vi "Version_2.0_Single_Column_Code.vi"() -> ()   [LabVIEW 2020] (continued)
                            # "Clean the tubing with Sample"
                            n4641 = local read "N-S"() -> (w5076:i32)
                            n4642 = for {
                              N: w5076 -> [_]
                              n4643 = stacked-sequence {
                                frame #0 {
                                n4644 = local read "VISA Refnum in\nfor Pump"() -> (w5079:refnum<visa-resource-name>)
                                n4645 = local read "Port for \nSample"() -> (w5078:string)
                                n4646 = call "PortChanger (SubVI).vi"("Port Number"=w5078, "VISA Refnum in"=w5079) -> ()  [unwired: 10 in]
                                }
                                frame #1 {
                                n4647 = local read "VISA Refnum in\nfor Pump"() -> (w5080:refnum<visa-resource-name>)
                                n4648 = call "ProcessCompletionWaiter (SubVI).vi"("VISA Refnum in"=w5080) -> ()  [unwired: 11 in]
                                }
                                frame #2 {
                                n4649 = local read "VISA Refnum in\nfor Pump"() -> (w5085:refnum<visa-resource-name>)
                                n4650 = local read "Sample PickUp \nFlow Rate (ul/min)"() -> (w5082:dbl)
                                n4651 = local read "V-S"() -> (w5081:dbl)
                                n4652 = local read "Volume of Syringe"() -> (w5083:dbl)
                                n4653 = call "RPickUp(SubVI).vi"("Volume to be picked up"=w5081, "Volume of Syringe"=w5083, "Resolution of PickUP"=T2."Standard Pumping", "PickUp Flow Rate (ul/min)"=w5082, "VISA Refnum in"=w5085) -> ()  [unwired: 6 in, 1 out]
                                }
                                frame #3 {
                                n4654 = local read "Stopper that ends \nthe main loops"() -> (w5086:bool)
                                n4655 = local read "VISA Refnum in\nfor Pump"() -> (w5087:refnum<visa-resource-name>)
                                n4656 = case shown="True" w5086 {
                                frame False {
                                }
                                frame True {
                                n4657 = local read "VISA Refnum in\nfor Pump"() -> (w5088:refnum<visa-resource-name>)
                                n4658 = call "HardStopCurrentProcess (SubVI).vi"("VISA Refnum in"=w5088) -> ()  [unwired: 11 in]
                                }
                                }
                                n4659 = call "ProcessCompletionWaiter (SubVI).vi"("VISA Refnum in"=w5087) -> ()  [unwired: 11 in]
                                }
                                frame #4 {
                                n4660 = local read "VISA Refnum in\nfor Pump"() -> (w5090:refnum<visa-resource-name>)
                                n4661 = call "PortChanger (SubVI).vi"("Port Number"="1", "VISA Refnum in"=w5090) -> ()  [unwired: 10 in]
                                }
                                frame #5 {
                                n4662 = local read "Stopper that ends \nthe main loops"() -> (w5091:bool)
                                n4663 = local read "VISA Refnum in\nfor Pump"() -> (w5092:refnum<visa-resource-name>)
                                n4664 = case shown="True" w5091 {
                                frame False {
                                }
                                frame True {
                                n4665 = local read "VISA Refnum in\nfor Pump"() -> (w5093:refnum<visa-resource-name>)
                                n4666 = call "HardStopCurrentProcess (SubVI).vi"("VISA Refnum in"=w5093) -> ()  [unwired: 11 in]
                                }
                                }
                                n4667 = call "ProcessCompletionWaiter (SubVI).vi"("VISA Refnum in"=w5092) -> ()  [unwired: 11 in]
                                }
                                frame #6 {
                                n4668 = local read "VISA Refnum in\nfor Pump"() -> (w5098:refnum<visa-resource-name>)
                                n4669 = local read "Volume of Syringe"() -> (w5095:dbl)
                                n4670 = call "GoToAbsolutePosition(SubVI).vi"("Absolute Volume Position in Syringe (in ul)"=0.0 ("Volume to be picked up"), "Volume of Syringe"=w5095, "Resolution of Pumping"=T2."Standard Pumping" ("Resolution of PickUP"), "Flow Rate (ul/min)"=150.0 ("PickUp Flow Rate (ul/min)"), "VISA Refnum in"=w5098) -> ()  [unwired: 6 in, 1 out]
                                }
                                frame #7 {
                                n4671 = local read "Stopper that ends \nthe main loops"() -> (w5099:bool)
                                n4672 = local read "VISA Refnum in\nfor Pump"() -> (w5100:refnum<visa-resource-name>)
                                n4673 = case shown="True" w5099 {
                                frame False {
                                }
                                frame True {
                                n4674 = local read "VISA Refnum in\nfor Pump"() -> (w5101:refnum<visa-resource-name>)
                                n4675 = call "HardStopCurrentProcess (SubVI).vi"("VISA Refnum in"=w5101) -> ()  [unwired: 11 in]
                                }
                                }
                                n4676 = call "ProcessCompletionWaiter (SubVI).vi"("VISA Refnum in"=w5100) -> ()  [unwired: 11 in]
                                }
                              }
                              n4677 = local write "Pause Data Collection"(TRUE ("Pause Data Collection")) -> ()
                            }
                          }
                        }
                      }
                      frame #1 {
                        # "Pump Sample into Column-1"
                        n4678 = stacked-sequence {
                          frame #0 {
                            # "Switch to Port-3"
                            # "Port-3 of pump is connected to Sample"
                            n4679 = local read "VISA Refnum in\nfor Pump"() -> (w5106:refnum<visa-resource-name>)
                            n4680 = local read "Port for \nSample"() -> (w5105:string)
                            n4681 = call "PortChanger (SubVI).vi"("Port Number"=w5105, "VISA Refnum in"=w5106) -> ()  [unwired: 10 in]
                          }
                          frame #1 {
                            n4682 = local read "VISA Refnum in\nfor Pump"() -> (w5107:refnum<visa-resource-name>)
                            n4683 = call "ProcessCompletionWaiter (SubVI).vi"("VISA Refnum in"=w5107) -> ()  [unwired: 11 in]
                          }
                          frame #2 {
                            n4684 = local write "Valve V1 Open"(TRUE ("Valve V1 Open")) -> ()
                            n4685 = local write "Valve V2 Open"(TRUE ("Valve V2 Open")) -> ()
                            n4686 = local write "Valve V3 Open"(FALSE ("Valve V3 Open")) -> ()
                            n4687 = local write "Valve V4 Open"(FALSE ("Valve V4 Open")) -> ()
                            n4688 = local write "External Valve \nOpen"(TRUE ("External Valve \nOpen")) -> ()
                            n4689 = local write "Valve V5 Open"(FALSE ("Valve V5 Open")) -> ()
                            n4690 = local write "Valve V8 Open"(FALSE ("Valve V8 Open")) -> ()
                            n4691 = local write "Valve V6 Open"(FALSE ("Valve V6 Open")) -> ()
                            n4692 = local write "Valve V7 Open"(FALSE ("Valve V7 Open")) -> ()
                          }
                          frame #3 {
                            n4693 = local read "Apparent Volume\nof Syringe"() -> (w5117:dbl)
                            n4694 = local read "Sample Volume \nto be Pumped"() -> (w5120:dbl)
                            n4695 = Quotient & Remainder(x=w5120, y=w5117) -> (x-y*floor(x/y)=w5118:dbl, floor(x/y)=w5119:dbl)
                            n4696 = for {
                              N: w5119 -> [_]
                              n4697 = stacked-sequence {
                                frame #0 {
                                n4698 = local read "Sample PickUp \nFlow Rate (ul/min)"() -> (w5123:dbl)
                                n4699 = local read "Sample Pumping\nResolution"() -> (w5122:T2)
                                n4700 = local read "VISA Refnum in\nfor Pump"() -> (w5125:refnum<visa-resource-name>)
                                n4701 = local read "Apparent Volume\nof Syringe"() -> (w5121:dbl)
                                n4702 = local read "Volume of Syringe"() -> (w5124:dbl)
                                n4703 = call "RPickUp(SubVI).vi"("Volume to be picked up"=w5121, "Volume of Syringe"=w5124, "Resolution of PickUP"=w5122, "PickUp Flow Rate (ul/min)"=w5123, "VISA Refnum in"=w5125) -> ()  [unwired: 6 in, 1 out]
                                }
                                frame #1 {
                                n4704 = local read "Stopper that ends \nthe main loops"() -> (w5126:bool)
                                n4705 = local read "VISA Refnum in\nfor Pump"() -> (w5127:refnum<visa-resource-name>)
                                n4706 = case shown="True" w5126 {
                                frame False {
                                }
                                frame True {
                                n4707 = local read "VISA Refnum in\nfor Pump"() -> (w5128:refnum<visa-resource-name>)
                                n4708 = call "HardStopCurrentProcess (SubVI).vi"("VISA Refnum in"=w5128) -> ()  [unwired: 11 in]
                                }
                                }
                                n4709 = call "ProcessCompletionWaiter (SubVI).vi"("VISA Refnum in"=w5127) -> ()  [unwired: 11 in]
                                }
                                frame #2 {
                                # "Reads the initial Plunger Position for computing the volume dispensed"
                                n4710 = local read "VISA Refnum in\nfor Pump"() -> (w5130:refnum<visa-resource-name>)
                                n4711 = call "AbsolutePlungerPosition (SubVI).vi"("VISA Refnum in"=w5130) -> ("Plunger Position"=w5129:i32)  [unwired: 10 in]
                                n4712 = local write "Initial Plunger Position"(w5129) -> ()
                                }
                                frame #3 {
                                # "Switch to Port-2"
                                # "Port-2 of the pump is conncted to column-1 of chip"
                                n4713 = local read "VISA Refnum in\nfor Pump"() -> (w5132:refnum<visa-resource-name>)
                                n4714 = call "PortChanger (SubVI).vi"("Port Number"="2", "VISA Refnum in"=w5132) -> ()  [unwired: 10 in]
                                }
                                frame #4 {
                                n4715 = local read "Stopper that ends \nthe main loops"() -> (w5133:bool)
                                n4716 = local read "VISA Refnum in\nfor Pump"() -> (w5134:refnum<visa-resource-name>)
                                n4717 = case shown="True" w5133 {
                                frame False {
                                }
                                frame True {
                                n4718 = local read "VISA Refnum in\nfor Pump"() -> (w5135:refnum<visa-resource-name>)
                                n4719 = call "HardStopCurrentProcess (SubVI).vi"("VISA Refnum in"=w5135) -> ()  [unwired: 11 in]
                                }
                                }
                                n4720 = call "ProcessCompletionWaiter (SubVI).vi"("VISA Refnum in"=w5134) -> ()  [unwired: 11 in]
                                }
                                frame #5 {
                                # "Keeps the AMF valve after column-1 open and valve after column-2 closed"
                                n4721 = local read "Sample Dispense\nFlow Rate (ul/min)"() -> (w5139:dbl)
                                n4722 = local read "Sample Pumping\nResolution"() -> (w5138:T2)
                                n4723 = local read "VISA Refnum in\nfor Pump"() -> (w5141:refnum<visa-resource-name>)
                                n4724 = local write "Pause Data Collection"(FALSE ("Pause Data Collection")) -> ()
                                n4725 = local read "Volume of Syringe"() -> (w5140:dbl)
                                n4726 = call "GoToAbsolutePosition(SubVI).vi"("Absolute Volume Position in Syringe (in ul)"=0.0 ("Volume to be Dispensed"), "Volume of Syringe"=w5140, "Resolution of Pumping"=w5138, "Flow Rate (ul/min)"=w5139, "VISA Refnum in"=w5141) -> ()  [unwired: 6 in, 1 out]
                                }
                                frame #6 {
                                n4727 = local read "Sample Pumping\nResolution"() -> (w5143:T2)
                                n4728 = local read "VISA Refnum in\nfor Pump"() -> (w5145:refnum<visa-resource-name>)
                                n4729 = local read "Initial Plunger Position"() -> (w5144:dbl)
                                n4730 = local read "Volume of Syringe"() -> (w5142:dbl)
                                n4731 = while {
                                tunnel: w5144 -> [w5152]
                                tunnel: w5145 -> [w5151]
                                tunnel: w5143 -> [w5150]
                                tunnel: w5142 -> [w5149]
                                stop <- w5147 stop-if-true
                                n4732 = stacked-sequence {
                                tunnel: w5152 -> [w5159 _]
                                tunnel: w5151 -> [w5158 w5179]
                                tunnel: w5150 -> [w5157 _]
                                tunnel: w5149 -> [w5156 _]
                                tunnel: [_ w5177] -> w5147
                                frame #0 {
                                n4733 = call "AbsolutePlungerPosition (SubVI).vi"("VISA Refnum in"=w5158) -> ("Plunger Position"=w5155:i32)  [unwired: 10 in]
                                n4734 = case shown="\"Standard Pumping\", Default" w5157 {
                                tunnel: w5159 -> [w5164 w5173]
                                tunnel: w5155 -> [w5165 w5172]
                                tunnel: [w5163 w5170] -> w5154
                                tunnel: w5156 -> [w5162 w5171]
                                frame "Standard Pumping", Default {
                                n4735 = Subtract(x=w5164, y=w5165) -> (x-y=w5161:dbl)
                                n4736 = Absolute Value(x=w5161) -> (abs(x)=w5160:dbl)
                                n4737 = Multiply(x=w5160, y=w5162) -> (x*y=w5167:dbl)
                                n4738 = Divide(x=w5167, y=3000.0) -> (x/y=w5163:dbl)
                                }
                                frame "High Resolution Pumping" {
                                n4739 = Subtract(x=w5173, y=w5172) -> (x-y=w5169:dbl)
                                n4740 = Absolute Value(x=w5169) -> (abs(x)=w5168:dbl)
                                n4741 = Multiply(x=w5168, y=w5171) -> (x*y=w5175:dbl)
                                n4742 = Divide(x=w5175, y=24000.0) -> (x/y=w5170:dbl)
                                }
                                }
                                n4743 = local write "Volume being Injected \nin this process"(w5154) -> ()
                                }
                                frame #1 {
                                n4744 = call "LSPOneStatus (SubVI).vi"("VISA Refnum in"=w5179) -> ("read buffer"=w5181:string)  [unwired: 10 in]
                                n4745 = call <vilib>:"Trim Whitespace.vi"("string"=w5181) -> ("trimmed string"=w5180:string)  [unwired: 1 in]
                                n4746 = local read "Stopper that ends \nthe main loops"() -> (w5176:bool)
                                n4747 = Equal?(x=w5180, y="/0`\u0003") -> (x = y?=w5178:bool)
                                n4748 = Or(x=w5178, y=w5176) -> (x .or. y?=w5177:bool)
                                }
                                }
                                n4749 = Wait (ms)(milliseconds to wait=u32 100) -> ()  [unwired: 1 out]
                                n4750 = local read "Stopper that ends \nthe main loops"() -> (w5146:bool)
                                n4751 = case shown="True" w5146 {
                                frame False {
                                }
                                frame True {
                                n4752 = local read "VISA Refnum in\nfor Pump"() -> (w5153:refnum<visa-resource-name>)
                                n4753 = call "HardStopCurrentProcess (SubVI).vi"("VISA Refnum in"=w5153) -> ()  [unwired: 11 in]
                                }
                                }
                                }
                                }
                                frame #7 {
                                # "Chnage the pump port back to Sample"
                                n4754 = local read "VISA Refnum in\nfor Pump"() -> (w5184:refnum<visa-resource-name>)
                                n4755 = local read "Port for \nSample"() -> (w5183:string)
                                n4756 = local write "Pause Data Collection"(TRUE ("Pause Data Collection")) -> ()
                                n4757 = Wait (ms)(milliseconds to wait=u32 500) -> ()  [unwired: 1 out]
                                n4758 = call "PortChanger (SubVI).vi"("Port Number"=w5183, "VISA Refnum in"=w5184) -> ()  [unwired: 10 in]
                                }
                                frame #8 {
                                n4759 = local read "VISA Refnum in\nfor Pump"() -> (w5187:refnum<visa-resource-name>)
                                n4760 = local write "Volume being Injected \nin this process"(0.0 ("Volume being Injected \nin this process")) -> ()
                                n4761 = call "ProcessCompletionWaiter (SubVI).vi"("VISA Refnum in"=w5187) -> ()  [unwired: 11 in]
                                }
                              }
                            }
                            n4762 = local write "Reminder of the \nVolume to be \nPumped"(w5118) -> ()
                          }
                          frame #4 {
                            n4763 = stacked-sequence {
                              frame #0 {
                                n4764 = local read "Sample PickUp \nFlow Rate (ul/min)"() -> (w5191:dbl)
                                n4765 = local read "Sample Pumping\nResolution"() -> (w5190:T2)
                                n4766 = local read "VISA Refnum in\nfor Pump"() -> (w5193:refnum<visa-resource-name>)
                                n4767 = local read "Reminder of the \nVolume to be \nPumped"() -> (w5189:dbl)
                                n4768 = local read "Volume of Syringe"() -> (w5192:dbl)
                                n4769 = call "RPickUp(SubVI).vi"("Volume to be picked up"=w5189, "Volume of Syringe"=w5192, "Resolution of PickUP"=w5190, "PickUp Flow Rate (ul/min)"=w5191, "VISA Refnum in"=w5193) -> ()  [unwired: 6 in, 1 out]
                              }
                              frame #1 {
                                n4770 = local read "Stopper that ends \nthe main loops"() -> (w5194:bool)
                                n4771 = local read "VISA Refnum in\nfor Pump"() -> (w5195:refnum<visa-resource-name>)
                                n4772 = case shown="True" w5194 {
                                frame False {
                                }
                                frame True {
                                n4773 = local read "VISA Refnum in\nfor Pump"() -> (w5196:refnum<visa-resource-name>)
                                n4774 = call "HardStopCurrentProcess (SubVI).vi"("VISA Refnum in"=w5196) -> ()  [unwired: 11 in]
                                }
                                }
                                n4775 = call "ProcessCompletionWaiter (SubVI).vi"("VISA Refnum in"=w5195) -> ()  [unwired: 11 in]
                              }
                              frame #2 {
                                # "Reads the initial Plunger Position for computing the volume dispensed"
                                n4776 = local read "VISA Refnum in\nfor Pump"() -> (w5198:refnum<visa-resource-name>)
                                n4777 = call "AbsolutePlungerPosition (SubVI).vi"("VISA Refnum in"=w5198) -> ("Plunger Position"=w5197:i32)  [unwired: 10 in]
                                n4778 = local write "Initial Plunger Position"(w5197) -> ()
                              }
                              frame #3 {
                                # "Switch to Port-2"
                                # "Port-2 of the pump is conncted to column-1 of chip"
                                n4779 = local read "VISA Refnum in\nfor Pump"() -> (w5200:refnum<visa-resource-name>)
                                n4780 = call "PortChanger (SubVI).vi"("Port Number"="2", "VISA Refnum in"=w5200) -> ()  [unwired: 10 in]
                              }
                              frame #4 {
                                n4781 = local read "Stopper that ends \nthe main loops"() -> (w5201:bool)
                                n4782 = local read "VISA Refnum in\nfor Pump"() -> (w5202:refnum<visa-resource-name>)
                                n4783 = case shown="True" w5201 {
                                frame False {
                                }
                                frame True {
                                n4784 = local read "VISA Refnum in\nfor Pump"() -> (w5203:refnum<visa-resource-name>)
                                n4785 = call "HardStopCurrentProcess (SubVI).vi"("VISA Refnum in"=w5203) -> ()  [unwired: 11 in]
                                }
                                }
                                n4786 = call "ProcessCompletionWaiter (SubVI).vi"("VISA Refnum in"=w5202) -> ()  [unwired: 11 in]
                              }
                              frame #5 {
                                # "Keeps the AMF valve after column-1 open and valve after column-2 closed"
                                n4787 = local read "Sample Dispense\nFlow Rate (ul/min)"() -> (w5207:dbl)
                                n4788 = local read "Sample Pumping\nResolution"() -> (w5206:T2)
                                n4789 = local read "VISA Refnum in\nfor Pump"() -> (w5209:refnum<visa-resource-name>)
                                n4790 = local write "Pause Data Collection"(FALSE ("Pause Data Collection")) -> ()
                                n4791 = local read "Volume of Syringe"() -> (w5208:dbl)
                                n4792 = call "GoToAbsolutePosition(SubVI).vi"("Absolute Volume Position in Syringe (in ul)"=0.0 ("Volume to be Dispensed"), "Volume of Syringe"=w5208, "Resolution of Pumping"=w5206, "Flow Rate (ul/min)"=w5207, "VISA Refnum in"=w5209) -> ()  [unwired: 6 in, 1 out]
                              }
                              frame #6 {
                                n4793 = local read "Sample Pumping\nResolution"() -> (w5211:T2)
                                n4794 = local read "VISA Refnum in\nfor Pump"() -> (w5213:refnum<visa-resource-name>)
                                n4795 = local read "Initial Plunger Position"() -> (w5212:dbl)
                                n4796 = local read "Volume of Syringe"() -> (w5210:dbl)
                                n4797 = while {
                                tunnel: w5212 -> [w5220]
                                tunnel: w5213 -> [w5219]
                                tunnel: w5211 -> [w5218]
                                tunnel: w5210 -> [w5217]
                                stop <- w5215 stop-if-true
                                n4798 = stacked-sequence {
                                tunnel: w5220 -> [w5227 _]
                                tunnel: w5219 -> [w5226 w5247]
                                tunnel: w5218 -> [w5225 _]
                                tunnel: w5217 -> [w5224 _]
                                tunnel: [_ w5245] -> w5215
                                frame #0 {
                                n4799 = call "AbsolutePlungerPosition (SubVI).vi"("VISA Refnum in"=w5226) -> ("Plunger Position"=w5223:i32)  [unwired: 10 in]
                                n4800 = case shown="\"Standard Pumping\", Default" w5225 {
                                tunnel: w5227 -> [w5232 w5241]
                                tunnel: w5223 -> [w5233 w5240]
                                tunnel: [w5231 w5238] -> w5222
                                tunnel: w5224 -> [w5230 w5239]
                                frame "Standard Pumping", Default {
                                n4801 = Subtract(x=w5232, y=w5233) -> (x-y=w5229:dbl)
                                n4802 = Absolute Value(x=w5229) -> (abs(x)=w5228:dbl)
                                n4803 = Multiply(x=w5228, y=w5230) -> (x*y=w5235:dbl)
                                n4804 = Divide(x=w5235, y=3000.0) -> (x/y=w5231:dbl)
                                }
                                frame "High Resolution Pumping" {
                                n4805 = Subtract(x=w5241, y=w5240) -> (x-y=w5237:dbl)
                                n4806 = Absolute Value(x=w5237) -> (abs(x)=w5236:dbl)
                                n4807 = Multiply(x=w5236, y=w5239) -> (x*y=w5243:dbl)
                                n4808 = Divide(x=w5243, y=24000.0) -> (x/y=w5238:dbl)
                                }
                                }
                                n4809 = local write "Volume being Injected \nin this process"(w5222) -> ()
                                }
                                frame #1 {
                                n4810 = call "LSPOneStatus (SubVI).vi"("VISA Refnum in"=w5247) -> ("read buffer"=w5249:string)  [unwired: 10 in]
                                n4811 = call <vilib>:"Trim Whitespace.vi"("string"=w5249) -> ("trimmed string"=w5248:string)  [unwired: 1 in]
                                n4812 = local read "Stopper that ends \nthe main loops"() -> (w5244:bool)
                                n4813 = Equal?(x=w5248, y="/0`\u0003") -> (x = y?=w5246:bool)
                                n4814 = Or(x=w5246, y=w5244) -> (x .or. y?=w5245:bool)
                                }
                                }
                                n4815 = Wait (ms)(milliseconds to wait=u32 100) -> ()  [unwired: 1 out]
                                n4816 = local read "Stopper that ends \nthe main loops"() -> (w5214:bool)
                                n4817 = case shown="True" w5214 {
                                frame False {
                                }
                                frame True {
                                n4818 = local read "VISA Refnum in\nfor Pump"() -> (w5221:refnum<visa-resource-name>)
                                n4819 = call "HardStopCurrentProcess (SubVI).vi"("VISA Refnum in"=w5221) -> ()  [unwired: 11 in]
                                }
                                }
                                }
                              }
                              frame #7 {
                                n4820 = local write "Pause Data Collection"(TRUE ("Pause Data Collection")) -> ()
                                n4821 = Wait (ms)(milliseconds to wait=u32 500) -> ()  [unwired: 1 out]
                              }
                              frame #8 {
                                n4822 = local write "Volume being Injected \nin this process"(0.0 ("Volume being Injected \nin this process")) -> ()
                              }
                            }
                          }
                        }
                        n4823 = local write "Equilibriating \nColumn-2"(FALSE ("Equilibriating \nColumn-2")) -> ()
                        n4824 = local write "Affinity On"(TRUE ("Affinity On")) -> ()
                        n4825 = local write "Sample pumping \ninto Column-1"(TRUE ("Sample pumping \ninto Column-1")) -> ()
                      }
                      frame #2 {
                        # "Wash Column-1 with Buffer-A2"
                        n4826 = local write "Sample pumping \ninto Column-1"(FALSE ("Sample pumping \ninto Column-1")) -> ()
                        n4827 = stacked-sequence {
                          frame #0 {
                            # "Switch to Port-4/6"
                            # "Port-4/6 of pump is connected to Buffer-A2"
                            n4828 = local read "VISA Refnum in\nfor Pump"() -> (w5257:refnum<visa-resource-name>)
                            n4829 = local read "Port for \nA2-Wash"() -> (w5256:string)
                            n4830 = call "PortChanger (SubVI).vi"("Port Number"=w5256, "VISA Refnum in"=w5257) -> ()  [unwired: 10 in]
                          }
                          frame #1 {
                            n4831 = local read "VISA Refnum in\nfor Pump"() -> (w5258:refnum<visa-resource-name>)
                            n4832 = call "ProcessCompletionWaiter (SubVI).vi"("VISA Refnum in"=w5258) -> ()  [unwired: 11 in]
                          }
                          frame #2 {
                            n4833 = local write "Valve V3 Open"(FALSE ("Valve V3 Open")) -> ()
                            n4834 = local write "Valve V4 Open"(FALSE ("Valve V4 Open")) -> ()
                            n4835 = local write "Valve V1 Open"(TRUE ("Valve V1 Open")) -> ()
                            n4836 = local write "Valve V2 Open"(TRUE ("Valve V2 Open")) -> ()
                            n4837 = local write "External Valve \nOpen"(TRUE ("Elution of Column-2")) -> ()
                            n4838 = local write "Valve V8 Open"(FALSE ("Valve V8 Open")) -> ()
                            n4839 = local write "Valve V5 Open"(FALSE ("Valve V5 Open")) -> ()
                            n4840 = local write "Valve V6 Open"(FALSE ("Valve V6 Open")) -> ()
                            n4841 = local write "Valve V7 Open"(FALSE ("Valve V7 Open")) -> ()
                          }
                          frame #3 {
                            n4842 = local read "Buffer-A2 Volume \nto be Pumped"() -> (w5271:dbl)
                            n4843 = local read "Apparent Volume\nof Syringe"() -> (w5268:dbl)
                            n4844 = Quotient & Remainder(x=w5271, y=w5268) -> (x-y*floor(x/y)=w5269:dbl, floor(x/y)=w5270:dbl)
                            n4845 = for {
                              N: w5270 -> [_]
                              n4846 = stacked-sequence {
                                frame #0 {
                                n4847 = local read "Buffer-A2 PickUp \nFlow Rate (ul/min)"() -> (w5274:dbl)
                                n4848 = local read "Buffer-A2 Pumping\nResolution"() -> (w5273:T2)
                                n4849 = local read "VISA Refnum in\nfor Pump"() -> (w5276:refnum<visa-resource-name>)
                                n4850 = local read "Apparent Volume\nof Syringe"() -> (w5272:dbl)
                                n4851 = local read "Volume of Syringe"() -> (w5275:dbl)
                                n4852 = call "RPickUp(SubVI).vi"("Volume to be picked up"=w5272, "Volume of Syringe"=w5275, "Resolution of PickUP"=w5273, "PickUp Flow Rate (ul/min)"=w5274, "VISA Refnum in"=w5276) -> ()  [unwired: 6 in, 1 out]
                                }
                                frame #1 {
                                n4853 = local read "Stopper that ends \nthe main loops"() -> (w5277:bool)
                                n4854 = local read "VISA Refnum in\nfor Pump"() -> (w5278:refnum<visa-resource-name>)
                                n4855 = case shown="True" w5277 {
                                frame False {
                                }
                                frame True {
                                n4856 = local read "VISA Refnum in\nfor Pump"() -> (w5279:refnum<visa-resource-name>)
                                n4857 = call "HardStopCurrentProcess (SubVI).vi"("VISA Refnum in"=w5279) -> ()  [unwired: 11 in]
                                }
                                }
                                n4858 = call "ProcessCompletionWaiter (SubVI).vi"("VISA Refnum in"=w5278) -> ()  [unwired: 11 in]
                                }
                                frame #2 {
                                # "Reads the initial Plunger Position for computing the volume dispensed"
                                n4859 = local read "VISA Refnum in\nfor Pump"() -> (w5281:refnum<visa-resource-name>)
                                n4860 = call "AbsolutePlungerPosition (SubVI).vi"("VISA Refnum in"=w5281) -> ("Plunger Position"=w5280:i32)  [unwired: 10 in]
                                n4861 = local write "Initial Plunger Position"(w5280) -> ()
                                }
                                frame #3 {
                                # "Switch to Port-2"
                                # "Port-2 of the pump is conncted to column-1 of chip"
                                n4862 = local read "VISA Refnum in\nfor Pump"() -> (w5283:refnum<visa-resource-name>)
                                n4863 = call "PortChanger (SubVI).vi"("Port Number"="2", "VISA Refnum in"=w5283) -> ()  [unwired: 10 in]
                                }
                                frame #4 {
                                n4864 = local read "Stopper that ends \nthe main loops"() -> (w5284:bool)
                                n4865 = local read "VISA Refnum in\nfor Pump"() -> (w5285:refnum<visa-resource-name>)
                                n4866 = case shown="True" w5284 {
                                frame False {
                                }
                                frame True {
                                n4867 = local read "VISA Refnum in\nfor Pump"() -> (w5286:refnum<visa-resource-name>)
                                n4868 = call "HardStopCurrentProcess (SubVI).vi"("VISA Refnum in"=w5286) -> ()  [unwired: 11 in]
                                }
                                }
                                n4869 = call "ProcessCompletionWaiter (SubVI).vi"("VISA Refnum in"=w5285) -> ()  [unwired: 11 in]
                                }
                                frame #5 {
                                # "Keeps the AMF valve after column-1 open and valve after column-2 closed"
                                n4870 = local read "Buffer-A2 Dispense\nFlow Rate (ul/min)"() -> (w5290:dbl)
                                n4871 = local read "Buffer-A2 Pumping\nResolution"() -> (w5289:T2)
                                n4872 = local read "VISA Refnum in\nfor Pump"() -> (w5292:refnum<visa-resource-name>)
                                n4873 = local write "Pause Data Collection"(FALSE ("Pause Data Collection")) -> ()
                                n4874 = local read "Volume of Syringe"() -> (w5291:dbl)
                                n4875 = call "GoToAbsolutePosition(SubVI).vi"("Absolute Volume Position in Syringe (in ul)"=0.0 ("Volume to be Dispensed"), "Volume of Syringe"=w5291, "Resolution of Pumping"=w5289, "Flow Rate (ul/min)"=w5290, "VISA Refnum in"=w5292) -> ()  [unwired: 6 in, 1 out]
                                }
                                frame #6 {
                                n4876 = local read "Buffer-A2 Pumping\nResolution"() -> (w5294:T2)
                                n4877 = local read "VISA Refnum in\nfor Pump"() -> (w5296:refnum<visa-resource-name>)
                                n4878 = local read "Initial Plunger Position"() -> (w5295:dbl)
                                n4879 = local read "Volume of Syringe"() -> (w5293:dbl)
                                n4880 = while {
                                tunnel: w5295 -> [w5303]
                                tunnel: w5296 -> [w5302]
                                tunnel: w5294 -> [w5301]
                                tunnel: w5293 -> [w5300]
                                stop <- w5298 stop-if-true
                                n4881 = stacked-sequence {
                                tunnel: w5303 -> [w5310 _]
                                tunnel: w5302 -> [w5309 w5330]
                                tunnel: w5301 -> [w5308 _]
                                tunnel: w5300 -> [w5307 _]
                                tunnel: [_ w5328] -> w5298
                                frame #0 {
                                n4882 = call "AbsolutePlungerPosition (SubVI).vi"("VISA Refnum in"=w5309) -> ("Plunger Position"=w5306:i32)  [unwired: 10 in]
                                n4883 = case shown="\"Standard Pumping\", Default" w5308 {
                                tunnel: w5310 -> [w5315 w5324]
                                tunnel: w5306 -> [w5316 w5323]
                                tunnel: [w5314 w5321] -> w5305
                                tunnel: w5307 -> [w5313 w5322]
                                frame "Standard Pumping", Default {
                                n4884 = Subtract(x=w5315, y=w5316) -> (x-y=w5312:dbl)
                                n4885 = Absolute Value(x=w5312) -> (abs(x)=w5311:dbl)
                                n4886 = Multiply(x=w5311, y=w5313) -> (x*y=w5318:dbl)
                                n4887 = Divide(x=w5318, y=3000.0) -> (x/y=w5314:dbl)
                                }
                                frame "High Resolution Pumping" {
                                n4888 = Subtract(x=w5324, y=w5323) -> (x-y=w5320:dbl)
                                n4889 = Absolute Value(x=w5320) -> (abs(x)=w5319:dbl)
                                n4890 = Multiply(x=w5319, y=w5322) -> (x*y=w5326:dbl)
                                n4891 = Divide(x=w5326, y=24000.0) -> (x/y=w5321:dbl)
                                }
                                }
                                n4892 = local write "Volume being Injected \nin this process"(w5305) -> ()
                                }
                                frame #1 {
                                n4893 = call "LSPOneStatus (SubVI).vi"("VISA Refnum in"=w5330) -> ("read buffer"=w5332:string)  [unwired: 10 in]
                                n4894 = call <vilib>:"Trim Whitespace.vi"("string"=w5332) -> ("trimmed string"=w5331:string)  [unwired: 1 in]
                                n4895 = local read "Stopper that ends \nthe main loops"() -> (w5327:bool)
                                n4896 = Equal?(x=w5331, y="/0`\u0003") -> (x = y?=w5329:bool)
                                n4897 = Or(x=w5329, y=w5327) -> (x .or. y?=w5328:bool)
                                }
                                }
                                n4898 = Wait (ms)(milliseconds to wait=u32 100) -> ()  [unwired: 1 out]
                                n4899 = local read "Stopper that ends \nthe main loops"() -> (w5297:bool)
                                n4900 = case shown="True" w5297 {
                                frame False {
                                }
                                frame True {
                                n4901 = local read "VISA Refnum in\nfor Pump"() -> (w5304:refnum<visa-resource-name>)
                                n4902 = call "HardStopCurrentProcess (SubVI).vi"("VISA Refnum in"=w5304) -> ()  [unwired: 11 in]
                                }
                                }
                                }
                                }
                                frame #7 {
                                # "Change the port back to Buffer-A2"
                                n4903 = local read "VISA Refnum in\nfor Pump"() -> (w5335:refnum<visa-resource-name>)
                                n4904 = local read "Port for \nA2-Wash"() -> (w5334:string)
                                n4905 = local write "Pause Data Collection"(TRUE ("Pause Data Collection")) -> ()
                                n4906 = Wait (ms)(milliseconds to wait=u32 500) -> ()  [unwired: 1 out]
                                n4907 = call "PortChanger (SubVI).vi"("Port Number"=w5334, "VISA Refnum in"=w5335) -> ()  [unwired: 10 in]
                                }
                                frame #8 {
                                n4908 = local read "VISA Refnum in\nfor Pump"() -> (w5338:refnum<visa-resource-name>)
                                n4909 = local write "Volume being Injected \nin this process"(0.0 ("Volume being Injected \nin this process")) -> ()
                                n4910 = call "ProcessCompletionWaiter (SubVI).vi"("VISA Refnum in"=w5338) -> ()  [unwired: 11 in]
                                }
                              }
                            }
                            n4911 = local write "Reminder of the \nVolume to be \nPumped"(w5269) -> ()
                          }
                          frame #4 {
                            n4912 = stacked-sequence {
                              frame #0 {
                                n4913 = local read "Buffer-A2 PickUp \nFlow Rate (ul/min)"() -> (w5342:dbl)
                                n4914 = local read "Buffer-A2 Pumping\nResolution"() -> (w5341:T2)
                                n4915 = local read "VISA Refnum in\nfor Pump"() -> (w5344:refnum<visa-resource-name>)
                                n4916 = local read "Reminder of the \nVolume to be \nPumped"() -> (w5340:dbl)
                                n4917 = local read "Volume of Syringe"() -> (w5343:dbl)
                                n4918 = call "RPickUp(SubVI).vi"("Volume to be picked up"=w5340, "Volume of Syringe"=w5343, "Resolution of PickUP"=w5341, "PickUp Flow Rate (ul/min)"=w5342, "VISA Refnum in"=w5344) -> ()  [unwired: 6 in, 1 out]
                              }
                              frame #1 {
                                n4919 = local read "Stopper that ends \nthe main loops"() -> (w5345:bool)
                                n4920 = local read "VISA Refnum in\nfor Pump"() -> (w5346:refnum<visa-resource-name>)
                                n4921 = case shown="True" w5345 {
                                frame False {
                                }
                                frame True {
                                n4922 = local read "VISA Refnum in\nfor Pump"() -> (w5347:refnum<visa-resource-name>)
                                n4923 = call "HardStopCurrentProcess (SubVI).vi"("VISA Refnum in"=w5347) -> ()  [unwired: 11 in]
                                }
                                }
                                n4924 = call "ProcessCompletionWaiter (SubVI).vi"("VISA Refnum in"=w5346) -> ()  [unwired: 11 in]
                              }
                              frame #2 {
                                # "Reads the initial Plunger Position for computing the volume dispensed"
                                n4925 = local read "VISA Refnum in\nfor Pump"() -> (w5349:refnum<visa-resource-name>)
                                n4926 = call "AbsolutePlungerPosition (SubVI).vi"("VISA Refnum in"=w5349) -> ("Plunger Position"=w5348:i32)  [unwired: 10 in]
                                n4927 = local write "Initial Plunger Position"(w5348) -> ()
                              }
                              frame #3 {
                                # "Switch to Port-2"
                                # "Port-2 of the pump is conncted to column-1 of chip"
                                n4928 = local read "VISA Refnum in\nfor Pump"() -> (w5351:refnum<visa-resource-name>)
                                n4929 = call "PortChanger (SubVI).vi"("Port Number"="2", "VISA Refnum in"=w5351) -> ()  [unwired: 10 in]
                              }
                              frame #4 {
                                n4930 = local read "Stopper that ends \nthe main loops"() -> (w5352:bool)
                                n4931 = local read "VISA Refnum in\nfor Pump"() -> (w5353:refnum<visa-resource-name>)
                                n4932 = case shown="True" w5352 {
                                frame False {
                                }
                                frame True {
                                n4933 = local read "VISA Refnum in\nfor Pump"() -> (w5354:refnum<visa-resource-name>)
                                n4934 = call "HardStopCurrentProcess (SubVI).vi"("VISA Refnum in"=w5354) -> ()  [unwired: 11 in]
                                }
                                }
                                n4935 = call "ProcessCompletionWaiter (SubVI).vi"("VISA Refnum in"=w5353) -> ()  [unwired: 11 in]
                              }
                              frame #5 {
                                # "Keeps the AMF valve after column-1 open and valve after column-2 closed"
                                n4936 = local read "Buffer-A2 Dispense\nFlow Rate (ul/min)"() -> (w5358:dbl)
                                n4937 = local read "Buffer-A2 Pumping\nResolution"() -> (w5357:T2)
                                n4938 = local read "VISA Refnum in\nfor Pump"() -> (w5360:refnum<visa-resource-name>)
                                n4939 = local write "Pause Data Collection"(FALSE ("Pause Data Collection")) -> ()
                                n4940 = local read "Volume of Syringe"() -> (w5359:dbl)
                                n4941 = call "GoToAbsolutePosition(SubVI).vi"("Absolute Volume Position in Syringe (in ul)"=0.0 ("Volume to be Dispensed"), "Volume of Syringe"=w5359, "Resolution of Pumping"=w5357, "Flow Rate (ul/min)"=w5358, "VISA Refnum in"=w5360) -> ()  [unwired: 6 in, 1 out]
                              }
                              frame #6 {
                                n4942 = local read "Buffer-A2 Pumping\nResolution"() -> (w5362:T2)
                                n4943 = local read "VISA Refnum in\nfor Pump"() -> (w5364:refnum<visa-resource-name>)
                                n4944 = local read "Initial Plunger Position"() -> (w5363:dbl)
                                n4945 = local read "Volume of Syringe"() -> (w5361:dbl)
                                n4946 = while {
                                tunnel: w5363 -> [w5371]
                                tunnel: w5364 -> [w5370]
                                tunnel: w5362 -> [w5369]
                                tunnel: w5361 -> [w5368]
                                stop <- w5366 stop-if-true
                                n4947 = stacked-sequence {
                                tunnel: w5371 -> [w5378 _]
                                tunnel: w5370 -> [w5377 w5398]
                                tunnel: w5369 -> [w5376 _]
                                tunnel: w5368 -> [w5375 _]
                                tunnel: [_ w5396] -> w5366
                                frame #0 {
                                n4948 = call "AbsolutePlungerPosition (SubVI).vi"("VISA Refnum in"=w5377) -> ("Plunger Position"=w5374:i32)  [unwired: 10 in]
                                n4949 = case shown="\"Standard Pumping\", Default" w5376 {
                                tunnel: w5378 -> [w5383 w5392]
                                tunnel: w5374 -> [w5384 w5391]
                                tunnel: [w5382 w5389] -> w5373
                                tunnel: w5375 -> [w5381 w5390]
                                frame "Standard Pumping", Default {
                                n4950 = Subtract(x=w5383, y=w5384) -> (x-y=w5380:dbl)
                                n4951 = Absolute Value(x=w5380) -> (abs(x)=w5379:dbl)
                                n4952 = Multiply(x=w5379, y=w5381) -> (x*y=w5386:dbl)
                                n4953 = Divide(x=w5386, y=3000.0) -> (x/y=w5382:dbl)
                                }
                                frame "High Resolution Pumping" {
                                n4954 = Subtract(x=w5392, y=w5391) -> (x-y=w5388:dbl)
                                n4955 = Absolute Value(x=w5388) -> (abs(x)=w5387:dbl)
                                n4956 = Multiply(x=w5387, y=w5390) -> (x*y=w5394:dbl)
                                n4957 = Divide(x=w5394, y=24000.0) -> (x/y=w5389:dbl)
                                }
                                }
                                n4958 = local write "Volume being Injected \nin this process"(w5373) -> ()
                                }
                                frame #1 {
                                n4959 = call "LSPOneStatus (SubVI).vi"("VISA Refnum in"=w5398) -> ("read buffer"=w5400:string)  [unwired: 10 in]
                                n4960 = call <vilib>:"Trim Whitespace.vi"("string"=w5400) -> ("trimmed string"=w5399:string)  [unwired: 1 in]
                                n4961 = local read "Stopper that ends \nthe main loops"() -> (w5395:bool)
                                n4962 = Equal?(x=w5399, y="/0`\u0003") -> (x = y?=w5397:bool)
                                n4963 = Or(x=w5397, y=w5395) -> (x .or. y?=w5396:bool)
                                }
                                }
                                n4964 = Wait (ms)(milliseconds to wait=u32 100) -> ()  [unwired: 1 out]
                                n4965 = local read "Stopper that ends \nthe main loops"() -> (w5365:bool)
                                n4966 = case shown="True" w5365 {
                                frame False {
                                }
                                frame True {
                                n4967 = local read "VISA Refnum in\nfor Pump"() -> (w5372:refnum<visa-resource-name>)
                                n4968 = call "HardStopCurrentProcess (SubVI).vi"("VISA Refnum in"=w5372) -> ()  [unwired: 11 in]
                                }
                                }
                                }
                              }
                              frame #7 {
                                n4969 = local write "Pause Data Collection"(TRUE ("Pause Data Collection")) -> ()
                                n4970 = Wait (ms)(milliseconds to wait=u32 500) -> ()  [unwired: 1 out]
                              }
                              frame #8 {
                                n4971 = local write "Volume being Injected \nin this process"(0.0 ("Volume being Injected \nin this process")) -> ()
                                n4972 = local write "Start the Process"(FALSE ("Start the Process")) -> ()
                              }
                            }
                          }
                        }
                        n4973 = local write "Washing Column-1"(TRUE ("Washing Column-1")) -> ()
                      }
                      frame #3 {
                        # "Connecting Buffer-C with port-5, cleaning the tubing with Buffer-C1, and washing the Column-2 to get rid of spill out from wash steps of column-1"
                        n4974 = local write "Washing Column-1"(FALSE ("Washing Column-1")) -> ()
                        n4975 = stacked-sequence {
                          frame #0 {
                            # "Switch to Port-5"
                            # "Port-5 of pump is connected to Buffer-C1"
                            n4976 = local read "VISA Refnum in\nfor Pump"() -> (w5409:refnum<visa-resource-name>)
                            n4977 = local read "Port for \nC1-Equilibriation"() -> (w5408:string)
                            n4978 = call "PortChanger (SubVI).vi"("Port Number"=w5408, "VISA Refnum in"=w5409) -> ()  [unwired: 10 in]
                          }
                          frame #1 {
                            n4979 = local read "VISA Refnum in\nfor Pump"() -> (w5410:refnum<visa-resource-name>)
                            n4980 = call "ProcessCompletionWaiter (SubVI).vi"("VISA Refnum in"=w5410) -> ()  [unwired: 11 in]
                          }
                          frame #2 {
                            # "Wash the inside of the pump valve"
                            n4981 = local read "n"() -> (w5411:i32)
                            n4982 = for {
                              N: w5411 -> [_]
                              n4983 = stacked-sequence {
                                frame #0 {
                                n4984 = local read "Buffer-A2 Pumping\nResolution"() -> (w5414:T2)
                                n4985 = local read "VISA Refnum in\nfor Pump"() -> (w5416:refnum<visa-resource-name>)
                                n4986 = local read "V-S"() -> (w5412:dbl)
                                n4987 = local read "Volume of Syringe"() -> (w5415:dbl)
                                n4988 = call "RPickUp(SubVI).vi"("Volume to be picked up"=w5412, "Volume of Syringe"=w5415, "Resolution of PickUP"=w5414, "PickUp Flow Rate (ul/min)"=150.0, "VISA Refnum in"=w5416) -> ()  [unwired: 6 in, 1 out]
                                }
                                frame #1 {
                                n4989 = local read "Stopper that ends \nthe main loops"() -> (w5417:bool)
                                n4990 = local read "VISA Refnum in\nfor Pump"() -> (w5418:refnum<visa-resource-name>)
                                n4991 = case shown="True" w5417 {
                                frame False {
                                }
                                frame True {
                                n4992 = local read "VISA Refnum in\nfor Pump"() -> (w5419:refnum<visa-resource-name>)
                                n4993 = call "HardStopCurrentProcess (SubVI).vi"("VISA Refnum in"=w5419) -> ()  [unwired: 11 in]
                                }
                                }
                                n4994 = call "ProcessCompletionWaiter (SubVI).vi"("VISA Refnum in"=w5418) -> ()  [unwired: 11 in]
                                }
                                frame #2 {
                                # "Switch to Port-1"
                                # "Port-1 of the pump is conncted to waste"
                                n4995 = local read "VISA Refnum in\nfor Pump"() -> (w5421:refnum<visa-resource-name>)
                                n4996 = call "PortChanger (SubVI).vi"("Port Number"="1", "VISA Refnum in"=w5421) -> ()  [unwired: 10 in]
                                }
                                frame #3 {
                                n4997 = local read "Stopper that ends \nthe main loops"() -> (w5422:bool)
                                n4998 = local read "VISA Refnum in\nfor Pump"() -> (w5423:refnum<visa-resource-name>)
                                n4999 = case shown="True" w5422 {
                                frame False {
                                }
                                frame True {
                                n5000 = local read "VISA Refnum in\nfor Pump"() -> (w5424:refnum<visa-resource-name>)
                                n5001 = call "HardStopCurrentProcess (SubVI).vi"("VISA Refnum in"=w5424) -> ()  [unwired: 11 in]
                                }
                                }
                                n5002 = call "ProcessCompletionWaiter (SubVI).vi"("VISA Refnum in"=w5423) -> ()  [unwired: 11 in]
                                }
                                frame #4 {
                                n5003 = local read "Buffer-A2 Pumping\nResolution"() -> (w5427:T2)
                                n5004 = local read "VISA Refnum in\nfor Pump"() -> (w5429:refnum<visa-resource-name>)
                                n5005 = local read "Volume of Syringe"() -> (w5428:dbl)
                                n5006 = call "GoToAbsolutePosition(SubVI).vi"("Absolute Volume Position in Syringe (in ul)"=0.0 ("Volume to be Dispensed"), "Volume of Syringe"=w5428, "Resolution of Pumping"=w5427, "Flow Rate (ul/min)"=150.0, "VISA Refnum in"=w5429) -> ()  [unwired: 6 in, 1 out]
                                }
                                frame #5 {
                                n5007 = local read "VISA Refnum in\nfor Pump"() -> (w5430:refnum<visa-resource-name>)
                                n5008 = call "ProcessCompletionWaiter (SubVI).vi"("VISA Refnum in"=w5430) -> ()  [unwired: 11 in]
                                }
                                frame #6 {
                                # "Change the port back to Buffer-C1"
                                n5009 = local read "VISA Refnum in\nfor Pump"() -> (w5432:refnum<visa-resource-name>)
                                n5010 = local read "Port for \nC1-Equilibriation"() -> (w5431:string)
                                n5011 = call "PortChanger (SubVI).vi"("Port Number"=w5431, "VISA Refnum in"=w5432) -> ()  [unwired: 10 in]
                                }
                                frame #7 {
                                n5012 = local read "VISA Refnum in\nfor Pump"() -> (w5433:refnum<visa-resource-name>)
                                n5013 = call "ProcessCompletionWaiter (SubVI).vi"("VISA Refnum in"=w5433) -> ()  [unwired: 11 in]
                                }
                              }
                            }
                          }
                          frame #3 {
                            # "Wash the pathway between column-2 and column-1 on chip"
                            n5014 = local read "n"() -> (w5434:i32)
                            n5015 = for {
                              N: w5434 -> [_]
                              n5016 = stacked-sequence {
                                frame #0 {
                                n5017 = local read "Buffer-A2 Pumping\nResolution"() -> (w5437:T2)
                                n5018 = local read "VISA Refnum in\nfor Pump"() -> (w5439:refnum<visa-resource-name>)
                                n5019 = local read "V-S"() -> (w5435:dbl)
                                n5020 = local read "Volume of Syringe"() -> (w5438:dbl)
                                n5021 = call "RPickUp(SubVI).vi"("Volume to be picked up"=w5435, "Volume of Syringe"=w5438, "Resolution of PickUP"=w5437, "PickUp Flow Rate (ul/min)"=150.0, "VISA Refnum in"=w5439) -> ()  [unwired: 6 in, 1 out]
                                }
                                frame #1 {
                                n5022 = local read "Stopper that ends \nthe main loops"() -> (w5440:bool)
                                n5023 = local read "VISA Refnum in\nfor Pump"() -> (w5441:refnum<visa-resource-name>)
                                n5024 = case shown="True" w5440 {
                                frame False {
                                }
                                frame True {
                                n5025 = local read "VISA Refnum in\nfor Pump"() -> (w5442:refnum<visa-resource-name>)
                                n5026 = call "HardStopCurrentProcess (SubVI).vi"("VISA Refnum in"=w5442) -> ()  [unwired: 11 in]
                                }
                                }
                                n5027 = call "ProcessCompletionWaiter (SubVI).vi"("VISA Refnum in"=w5441) -> ()  [unwired: 11 in]
                                }
                                frame #2 {
                                # "Switch to Port-10"
                                # "Port-10 of the pump is conncted to column-2"
                                n5028 = local read "VISA Refnum in\nfor Pump"() -> (w5444:refnum<visa-resource-name>)
                                n5029 = call "PortChanger (SubVI).vi"("Port Number"="10", "VISA Refnum in"=w5444) -> ()  [unwired: 10 in]
                                }
                                frame #3 {
                                n5030 = local read "Stopper that ends \nthe main loops"() -> (w5445:bool)
                                n5031 = local read "VISA Refnum in\nfor Pump"() -> (w5446:refnum<visa-resource-name>)
                                n5032 = case shown="True" w5445 {
                                frame False {
                                }
                                frame True {
                                n5033 = local read "VISA Refnum in\nfor Pump"() -> (w5447:refnum<visa-resource-name>)
                                n5034 = call "HardStopCurrentProcess (SubVI).vi"("VISA Refnum in"=w5447) -> ()  [unwired: 11 in]
                                }
                                }
                                n5035 = call "ProcessCompletionWaiter (SubVI).vi"("VISA Refnum in"=w5446) -> ()  [unwired: 11 in]
                                }
                                frame #4 {
                                n5036 = local read "Buffer-A2 Pumping\nResolution"() -> (w5455:T2)
                                n5037 = local read "VISA Refnum in\nfor Pump"() -> (w5457:refnum<visa-resource-name>)
                                n5038 = local read "f"() -> (w5449:dbl)
                                n5039 = local read "Volume of Syringe"() -> (w5456:dbl)
                                n5040 = call "GoToAbsolutePosition(SubVI).vi"("Absolute Volume Position in Syringe (in ul)"=0.0 ("Volume to be Dispensed"), "Volume of Syringe"=w5456, "Resolution of Pumping"=w5455, "Flow Rate (ul/min)"=w5449, "VISA Refnum in"=w5457) -> ()  [unwired: 6 in, 1 out]
                                n5041 = local write "External Valve \nOpen"(TRUE ("External Valve \nOpen")) -> ()
                                n5042 = local write "Valve V2 Open"(TRUE ("Valve V2 Open")) -> ()
                                n5043 = local write "Valve V1 Open"(FALSE ("Valve V1 Open")) -> ()
                                n5044 = local write "Valve V4 Open"(FALSE ("Valve V4 Open")) -> ()
                                n5045 = local write "Valve V3 Open"(TRUE ("Valve V3 Open")) -> ()
                                }
                                frame #5 {
                                n5046 = local read "VISA Refnum in\nfor Pump"() -> (w5458:refnum<visa-resource-name>)
                                n5047 = call "ProcessCompletionWaiter (SubVI).vi"("VISA Refnum in"=w5458) -> ()  [unwired: 11 in]
                                }
                                frame #6 {
                                # "Change the port back to Buffer-C1"
                                n5048 = local read "VISA Refnum in\nfor Pump"() -> (w5460:refnum<visa-resource-name>)
                                n5049 = local read "Port for \nC1-Equilibriation"() -> (w5459:string)
                                n5050 = call "PortChanger (SubVI).vi"("Port Number"=w5459, "VISA Refnum in"=w5460) -> ()  [unwired: 10 in]
                                }
                                frame #7 {
                                n5051 = local read "VISA Refnum in\nfor Pump"() -> (w5461:refnum<visa-resource-name>)
                                n5052 = call "ProcessCompletionWaiter (SubVI).vi"("VISA Refnum in"=w5461) -> ()  [unwired: 11 in]
                                }
                              }
                            }
                          }
                          frame #4 {
                            # "Washes the SEC column"
                            n5053 = local read "Apparent Volume\nof Syringe"() -> (w5464:dbl)
                            n5054 = local read "c"() -> (w5465:dbl)
                            n5055 = Quotient & Remainder(x=w5465, y=w5464) -> (x-y*floor(x/y)=w5463:dbl, floor(x/y)=w5462:dbl)
                            n5056 = for {
                              N: w5462 -> [_]
                              n5057 = stacked-sequence {
                                frame #0 {
                                n5058 = local read "Buffer-A2 Pumping\nResolution"() -> (w5468:T2)
                                n5059 = local read "VISA Refnum in\nfor Pump"() -> (w5470:refnum<visa-resource-name>)
                                n5060 = local read "Apparent Volume\nof Syringe"() -> (w5466:dbl)
                                n5061 = local read "Volume of Syringe"() -> (w5469:dbl)
                                n5062 = call "RPickUp(SubVI).vi"("Volume to be picked up"=w5466, "Volume of Syringe"=w5469, "Resolution of PickUP"=w5468, "PickUp Flow Rate (ul/min)"=150.0, "VISA Refnum in"=w5470) -> ()  [unwired: 6 in, 1 out]
                                }
                                frame #1 {
                                n5063 = local read "Stopper that ends \nthe main loops"() -> (w5471:bool)
                                n5064 = local read "VISA Refnum in\nfor Pump"() -> (w5472:refnum<visa-resource-name>)
                                n5065 = case shown="True" w5471 {
                                frame False {
                                }
                                frame True {
                                n5066 = local read "VISA Refnum in\nfor Pump"() -> (w5473:refnum<visa-resource-name>)
                                n5067 = call "HardStopCurrentProcess (SubVI).vi"("VISA Refnum in"=w5473) -> ()  [unwired: 11 in]
                                }
                                }
                                n5068 = call "ProcessCompletionWaiter (SubVI).vi"("VISA Refnum in"=w5472) -> ()  [unwired: 11 in]
                                }
                                frame #2 {
                                # "Switch to Port-10"
                                # "Port-10 of the pump is conncted to column-2 of chip"
                                n5069 = local read "VISA Refnum in\nfor Pump"() -> (w5475:refnum<visa-resource-name>)
                                n5070 = call "PortChanger (SubVI).vi"("Port Number"="10", "VISA Refnum in"=w5475) -> ()  [unwired: 10 in]
                                }
                                frame #3 {
                                n5071 = local read "Stopper that ends \nthe main loops"() -> (w5476:bool)
                                n5072 = local read "VISA Refnum in\nfor Pump"() -> (w5477:refnum<visa-resource-name>)
                                n5073 = case shown="True" w5476 {
                                frame False {
                                }
                                frame True {
                                n5074 = local read "VISA Refnum in\nfor Pump"() -> (w5478:refnum<visa-resource-name>)
                                n5075 = call "HardStopCurrentProcess (SubVI).vi"("VISA Refnum in"=w5478) -> ()  [unwired: 11 in]
                                }
                                }
                                n5076 = call "ProcessCompletionWaiter (SubVI).vi"("VISA Refnum in"=w5477) -> ()  [unwired: 11 in]
                                }
                                frame #4 {
                                # "Keeps the AMF valve after column-1 open and valve after column-2 closed"
                                n5077 = local read "Buffer-A2 Pumping\nResolution"() -> (w5490:T2)
                                n5078 = local read "VISA Refnum in\nfor Pump"() -> (w5492:refnum<visa-resource-name>)
                                n5079 = local read "f"() -> (w5484:dbl)
                                n5080 = local write "Valve V3 Open"(TRUE ("Valve V3 Open")) -> ()
                                n5081 = local write "Valve V2 Open"(FALSE ("Valve V2 Open")) -> ()
                                n5082 = local write "Valve V4 Open"(TRUE ("Valve V4 Open")) -> ()
                                n5083 = local write "Valve V1 Open"(FALSE ("Valve V1 Open")) -> ()
                                n5084 = local read "Volume of Syringe"() -> (w5491:dbl)
                                n5085 = call "GoToAbsolutePosition(SubVI).vi"("Absolute Volume Position in Syringe (in ul)"=0.0 ("Volume to be Dispensed"), "Volume of Syringe"=w5491, "Resolution of Pumping"=w5490, "Flow Rate (ul/min)"=w5484, "VISA Refnum in"=w5492) -> ()  [unwired: 6 in, 1 out]
                                n5086 = local write "External Valve \nOpen"(FALSE ("External Valve \nOpen")) -> ()
                                n5087 = local write "Valve V8 Open"(FALSE ("Valve V8 Open")) -> ()
                                n5088 = local write "Valve V5 Open"(TRUE ("Valve V5 Open")) -> ()
                                n5089 = local write "Valve V6 Open"(FALSE ("Valve V6 Open")) -> ()
                                n5090 = local write "Valve V7 Open"(TRUE ("Valve V7 Open")) -> ()
                                }
                                frame #5 {
                                n5091 = local read "VISA Refnum in\nfor Pump"() -> (w5493:refnum<visa-resource-name>)
                                n5092 = call "ProcessCompletionWaiter (SubVI).vi"("VISA Refnum in"=w5493) -> ()  [unwired: 11 in]
                                }
                                frame #6 {
                                # "Change the port back to Buffer-C1"
                                n5093 = local read "VISA Refnum in\nfor Pump"() -> (w5495:refnum<visa-resource-name>)
                                n5094 = local read "Port for \nC1-Equilibriation"() -> (w5494:string)
                                n5095 = call "PortChanger (SubVI).vi"("Port Number"=w5494, "VISA Refnum in"=w5495) -> ()  [unwired: 10 in]
                                }
                                frame #7 {
                                n5096 = local read "VISA Refnum in\nfor Pump"() -> (w5496:refnum<visa-resource-name>)
                                n5097 = call "ProcessCompletionWaiter (SubVI).vi"("VISA Refnum in"=w5496) -> ()  [unwired: 11 in]
                                }
                              }
                            }
                            n5098 = local write "Reminder of the \nVolume to be \nPumped"(w5463) -> ()
                          }
                          frame #5 {
                            # "Washes the SEC column"
                            n5099 = stacked-sequence {
                              frame #0 {
                                n5100 = local read "Buffer-A2 Pumping\nResolution"() -> (w5499:T2)
                                n5101 = local read "VISA Refnum in\nfor Pump"() -> (w5501:refnum<visa-resource-name>)
                                n5102 = local read "Reminder of the \nVolume to be \nPumped"() -> (w5497:dbl)
                                n5103 = local read "Volume of Syringe"() -> (w5500:dbl)
                                n5104 = call "RPickUp(SubVI).vi"("Volume to be picked up"=w5497, "Volume of Syringe"=w5500, "Resolution of PickUP"=w5499, "PickUp Flow Rate (ul/min)"=150.0, "VISA Refnum in"=w5501) -> ()  [unwired: 6 in, 1 out]
                              }
                              frame #1 {
                                n5105 = local read "Stopper that ends \nthe main loops"() -> (w5502:bool)
                                n5106 = local read "VISA Refnum in\nfor Pump"() -> (w5503:refnum<visa-resource-name>)
                                n5107 = case shown="True" w5502 {
                                frame False {
                                }
                                frame True {
                                n5108 = local read "VISA Refnum in\nfor Pump"() -> (w5504:refnum<visa-resource-name>)
                                n5109 = call "HardStopCurrentProcess (SubVI).vi"("VISA Refnum in"=w5504) -> ()  [unwired: 11 in]
                                }
                                }
                                n5110 = call "ProcessCompletionWaiter (SubVI).vi"("VISA Refnum in"=w5503) -> ()  [unwired: 11 in]
                              }
                              frame #2 {
                                # "Switch to Port-10"
                                # "Port-10 of the pump is conncted to column-2 of chip"
                                n5111 = local read "VISA Refnum in\nfor Pump"() -> (w5506:refnum<visa-resource-name>)
                                n5112 = call "PortChanger (SubVI).vi"("Port Number"="10", "VISA Refnum in"=w5506) -> ()  [unwired: 10 in]
                              }
                              frame #3 {
                                n5113 = local read "Stopper that ends \nthe main loops"() -> (w5507:bool)
                                n5114 = local read "VISA Refnum in\nfor Pump"() -> (w5508:refnum<visa-resource-name>)
                                n5115 = case shown="True" w5507 {
                                frame False {
                                }
                                frame True {
                                n5116 = local read "VISA Refnum in\nfor Pump"() -> (w5509:refnum<visa-resource-name>)
                                n5117 = call "HardStopCurrentProcess (SubVI).vi"("VISA Refnum in"=w5509) -> ()  [unwired: 11 in]
                                }
                                }
                                n5118 = call "ProcessCompletionWaiter (SubVI).vi"("VISA Refnum in"=w5508) -> ()  [unwired: 11 in]
                              }
                              frame #4 {
                                n5119 = local read "Buffer-A2 Pumping\nResolution"() -> (w5521:T2)
                                n5120 = local read "VISA Refnum in\nfor Pump"() -> (w5523:refnum<visa-resource-name>)
                                n5121 = local read "f"() -> (w5515:dbl)
                                n5122 = local read "Volume of Syringe"() -> (w5522:dbl)
                                n5123 = call "GoToAbsolutePosition(SubVI).vi"("Absolute Volume Position in Syringe (in ul)"=0.0 ("Volume to be Dispensed"), "Volume of Syringe"=w5522, "Resolution of Pumping"=w5521, "Flow Rate (ul/min)"=w5515, "VISA Refnum in"=w5523) -> ()  [unwired: 6 in, 1 out]
                                n5124 = local write "Valve V3 Open"(TRUE ("Valve V3 Open")) -> ()
                                n5125 = local write "Valve V2 Open"(FALSE ("Valve V2 Open")) -> ()
                                n5126 = local write "Valve V1 Open"(FALSE ("Valve V1 Open")) -> ()
                                n5127 = local write "Valve V4 Open"(TRUE ("Valve V4 Open")) -> ()
                                n5128 = local write "External Valve \nOpen"(FALSE ("External Valve \nOpen")) -> ()
                                n5129 = local write "Valve V8 Open"(FALSE ("Valve V8 Open")) -> ()
                                n5130 = local write "Valve V6 Open"(TRUE ("Valve V6 Open")) -> ()
                                n5131 = local write "Valve V5 Open"(TRUE ("Valve V5 Open")) -> ()
                                n5132 = local write "Valve V7 Open"(TRUE ("Valve V7 Open")) -> ()
                              }
                              frame #5 {
                                n5133 = local read "VISA Refnum in\nfor Pump"() -> (w5524:refnum<visa-resource-name>)
                                n5134 = call "ProcessCompletionWaiter (SubVI).vi"("VISA Refnum in"=w5524) -> ()  [unwired: 11 in]
                              }
                            }
                          }
                        }
                        n5135 = local write "Washing Column-2"(TRUE ("Washing Column-2")) -> ()
                      }
                      frame #4 {
                        # "Elute Column-1, Divert Sample into Column-2, Elute column-2 and Divert the sample onto Grid"
                        n5136 = stacked-sequence {
                          frame #0 {
                            # "Switch to Port-7"
                            # "Port-7 of pump is connected to Buffer-B"
                            n5137 = local write "Washing Column-2"(FALSE ("Washing Column-2")) -> ()
                            n5138 = local read "VISA Refnum in\nfor Pump"() -> (w5529:refnum<visa-resource-name>)
                            n5139 = local read "Port for \nB-Elution"() -> (w5527:string)
                            n5140 = local write "Affinity Elution On"(TRUE ("Affinity Elution On")) -> ()
                            n5141 = call "PortChanger (SubVI).vi"("Port Number"=w5527, "VISA Refnum in"=w5529) -> ()  [unwired: 10 in]
                            n5142 = local write "Elution of Column-1"(TRUE ("Elution of Column-1")) -> ()
                          }
                          frame #1 {
                            n5143 = local read "VISA Refnum in\nfor Pump"() -> (w5530:refnum<visa-resource-name>)
                            n5144 = call "ProcessCompletionWaiter (SubVI).vi"("VISA Refnum in"=w5530) -> ()  [unwired: 11 in]
                          }
                          frame #2 {
                            # "If Yes, it will clean the elution buffer from port-5 tubing a bit more"
                            n5145 = stacked-sequence {
                              frame #0 {
                                n5146 = local read "Buffer-B Pumping\nResolution"() -> (w5533:T2)
                                n5147 = local read "VISA Refnum in\nfor Pump"() -> (w5535:refnum<visa-resource-name>)
                                n5148 = local read "V-S"() -> (w5532:dbl)
                                n5149 = local read "Volume of Syringe"() -> (w5534:dbl)
                                n5150 = call "RPickUp(SubVI).vi"("Volume to be picked up"=w5532, "Volume of Syringe"=w5534, "Resolution of PickUP"=w5533, "PickUp Flow Rate (ul/min)"=150.0, "VISA Refnum in"=w5535) -> ()  [unwired: 6 in, 1 out]
                              }
                              frame #1 {
                                n5151 = local read "Stopper that ends \nthe main loops"() -> (w5536:bool)
                                n5152 = local read "VISA Refnum in\nfor Pump"() -> (w5537:refnum<visa-resource-name>)
                                n5153 = case shown="True" w5536 {
                                frame False {
                                }
                                frame True {
                                n5154 = local read "VISA Refnum in\nfor Pump"() -> (w5538:refnum<visa-resource-name>)
                                n5155 = call "HardStopCurrentProcess (SubVI).vi"("VISA Refnum in"=w5538) -> ()  [unwired: 11 in]
                                }
                                }
                                n5156 = call "ProcessCompletionWaiter (SubVI).vi"("VISA Refnum in"=w5537) -> ()  [unwired: 11 in]
                              }
